vi "Write Allow dropping.vi"(5 "Allow dropping":bool, 9 "Path in":refnum<class "Path.lvclass">) -> (3 "Path out":refnum<class "Path.lvclass">)   [LabVIEW 2014, in "Path.lvclass"]
uses:
  Path.lvclass
  Path.lvclass/Path.ctl
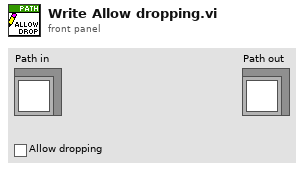
[diagram p1: front panel]
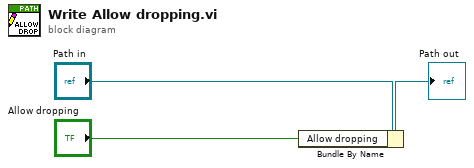
[diagram p0: block diagram]
diagram:
  n1 = Bundle By Name(cluster="Path in", "Allow dropping"="Allow dropping") -> (→"Path out":refnum<class "Path.lvclass">)
